vi "Remove value from array.vi"(8 "Value to remove":dbl, 11 "Input array":dbl[](graph)) -> (0 "Length reduction":i32, 3 "Output array":dbl[](graph))   [LabVIEW 2018]
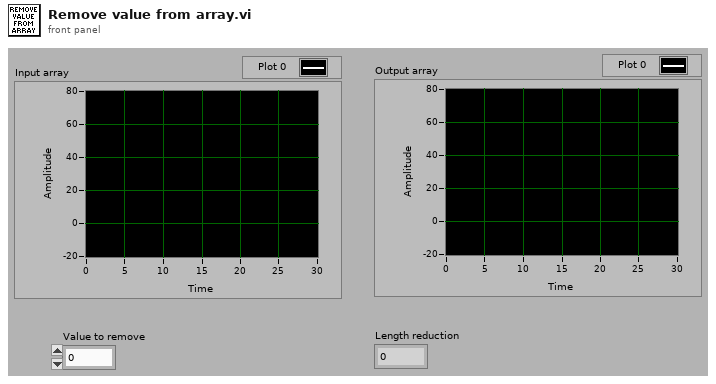
[diagram p1: front panel]
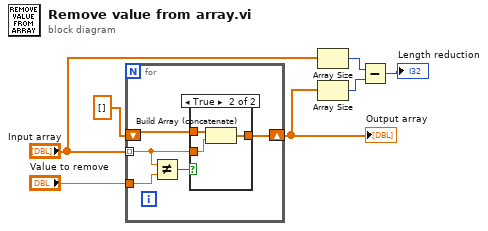
[diagram p0: block diagram]
diagram:
  n1 = for {
    tunnel: "Input array" -> [w10] mode=indexing
    shift-right: [w12] -> w4
    shift-left: dbl[] [] -> [w11]
    tunnel: "Value to remove" -> [w9]
    n2 = Not Equal?(x=w10, y=w9) -> (x != y?=w8:bool)
    n3 = case shown="True" w8 {
      tunnel: w10 -> [_ w16]
      tunnel: [w13 w15] -> w12
      tunnel: w11 -> [w13 w14]
      frame False {
      }
      frame True {
        n4 = Build Array (concatenate)(w14, w16) -> (w15:dbl[])
      }
    }
  }
  "Output array" <- w4
  n5 = Array Size(array="Input array") -> (size(s)=w2:i32)
  n6 = Array Size(array=w4) -> (size(s)=w3:i32)
  n7 = Subtract(x=w2, y=w3) -> (x-y=→"Length reduction":i32)
